vi "TSM Set DAQmx PSR Tasks.vi"(0 "TSM context":T1, 1 "max V":dbl=10.0 format="%0.2f", 5 "Sampling Rate (Hz)":dbl=1000.0 format="%#_6pHz", 7 "samples per channel":i32=1000, 11 "error in (no error)":errorcluster, 12 "min V":dbl=-10.0 format="%0.2f") -> (15 "error out":errorcluster)   [LabVIEW 2020]
doc: "Use this VI to initialize AI and AO tasks for all NI-DAQmx instruments in the pin map associated with the test program."
uses:
  <vilib>/NI_TestStand_SemiconductorModule/NI_TestStand_Semiconductor_Module.lvlibp/PinMap/General/SemiconductorModuleContext.ctl
  <vilib>/DAQmx/create/channels.llb/DAQmx Create Channel (AO-Voltage-Basic).vi
  <vilib>/DAQmx/configure/timing.llb/DAQmx Timing (Sample Clock).vi
  <vilib>/NI_TestStand_SemiconductorModule/NI_TestStand_Semiconductor_Module.lvlibp
  <resource>/objmgr/daqmx.rc
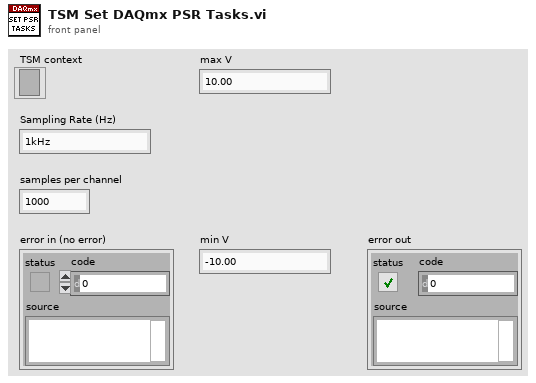
[diagram p1: front panel]
types:
  T1 = typedef "NI_TestStand_Semiconductor_Module.lvlibp/SemiconductorModuleContext.ctl" = refnum<k7>
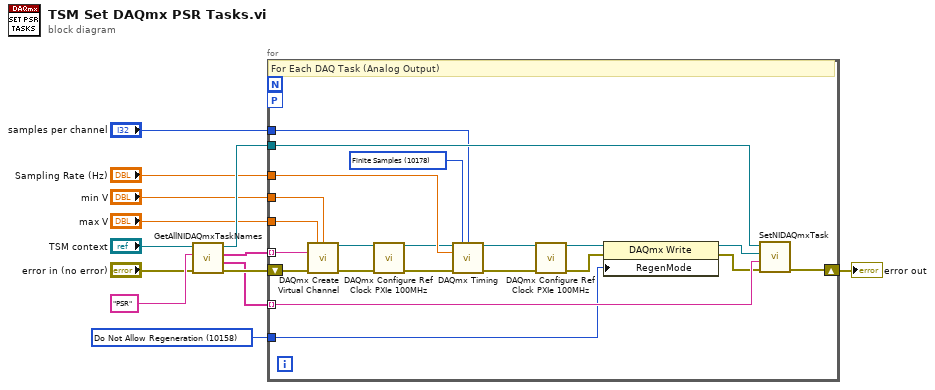
[diagram p0: block diagram]
diagram:
  w2 = 10158 items=["Allow Regeneration"=10097, "Do Not Allow Regeneration"=10158] ("RegenMode")
  n1 = call <vilib>:"GetAllNIDAQmxTaskNames.vi"("error in (no error)"="error in (no error)", "Task Type"="PSR", "Semiconductor Module Context"="TSM context") -> ("error out"=w12:errorcluster, "Task Names"=w11:string[], "Channel Lists"=w10:string[], "Semiconductor Module Context Out"=w13:T1)  [unwired: 5 in]
  n2 = for {
    tunnel: w13 -> [w33]
    tunnel: w11 -> [w30] mode=indexing
    tunnel: w10 -> [w31] mode=indexing
    shift-right: [w32] -> w6
    shift-left: w12 -> [w34]
    tunnel: "Sampling Rate (Hz)" -> [w25]
    tunnel: "max V" -> [w20]
    tunnel: "min V" -> [w19]
    tunnel: w2 -> [w18]
    workers-P: _ -> [_]
    tunnel: "samples per channel" -> [w14]
    w29 = 10178 items=["Finite Samples"=10178, "Continuous Samples"=10123, "Hardware Timed Single Point"=12522] ("sample mode")
    # "For Each DAQ Task (Analog Output)"
    n3 = call-poly <vilib>:"DAQmx Create Virtual Channel.vi"("maximum value"=w20, "minimum value"=w19, "physical channels"=w31, "error in"=w34) -> ("task out"=w24:refnum<k21>, "error out"=w23:errorcluster)  [unwired: 10 in]
    n4 = call "DAQmx Configure Ref Clock PXIe 100MHz.vi"("DAQmx Task In"=w24, "error in (no error)"=w23) -> ("DAQmx Task Out"=w22:refnum<k21>, "error out"=w21:errorcluster)  [unwired: 12 in]
    n5 = call-poly <vilib>:"DAQmx Timing.vi"("task/channels in"=w22, "sample mode"=w29, "samples per channel"=w14, "rate"=w25, "error in"=w21) -> ("task out"=w16:refnum<k21>, "error out"=w28:errorcluster)  [unwired: 9 in]
    n6 = call "DAQmx Configure Ref Clock PXIe 100MHz.vi"("DAQmx Task In"=w16, "error in (no error)"=w28) -> ("DAQmx Task Out"=w15:refnum<k21>, "error out"=w17:errorcluster)  [unwired: 12 in]
    n7 = property class="DAQmx Write"(reference=w15, error in=w17, "RegenMode"=w18) -> (reference out=w27:refnum<k21>, error out=w26:errorcluster)
    n8 = call <vilib>:"SetNIDAQmxTask.vi"("error in (no error)"=w26, "Task Name"=w30, "DAQmx Task"=w27, "Semiconductor Module Context"=w33) -> ("error out"=w32:errorcluster)  [unwired: 6 in, 1 out]
  }
  "error out" <- w6
